vi "Detect Platform Compatiblity.vi"(11 "Filename":string) -> (3 "Compatible":bool)   [LabVIEW 2011]
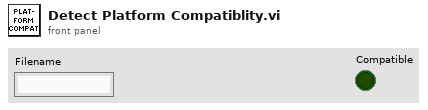
[diagram p1: front panel]
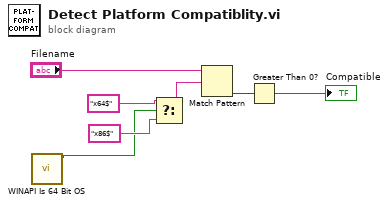
[diagram p0: block diagram]
diagram:
  n1 = call "WINAPI Is 64 Bit OS.vi"() -> ("Is64Bit"=w1:bool)  [unwired: 10 in, 1 out]
  n2 = Select(t="x64$" ("regular expression"), s=w1, f="x86$" ("regular expression")) -> (s? t:f=w4:string)
  n3 = Match Pattern(string="Filename", regular expression=w4) -> (offset past match=w6:i32)  [unwired: 1 in, 3 out]
  n4 = Greater Than 0?(x=w6) -> (x > 0?=→"Compatible":bool)
